vi "ALTS-2015 _Safety Logic LV2GBL.vi"(7 "Options":T1, 8 "error in (no error)":errorcluster, 10 "EStop In":bool) -> (0 "error out":errorcluster, 1 "S/W EStop":bool, 2 "EStop Out":bool, 3 "H/W EStop":bool)   [LabVIEW 2013]
uses:
  Controls/ALTS-2015 Safety Logic Cases.ctl
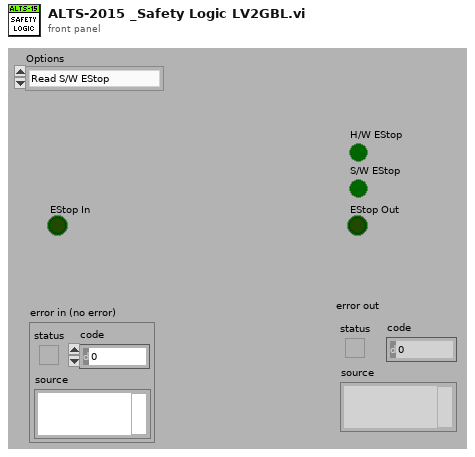
[diagram p1: front panel]
types:
  T1 = typedef "ALTS-2015 Safety Logic Cases.ctl" = enum16{"Read S/W EStop", "Read H/W EStop", "Write S/W EStop", "Write H/W EStop", "Read S/W & H/W EStop"}
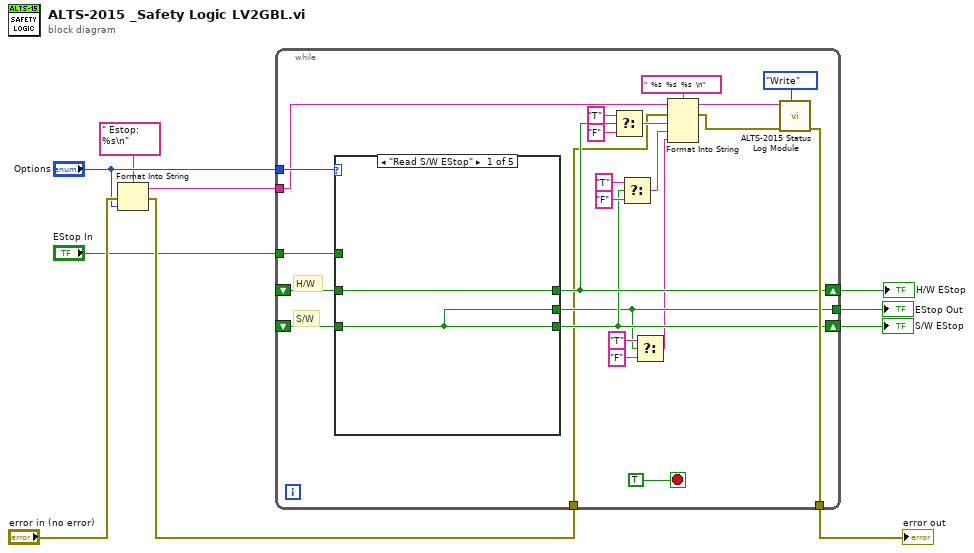
[diagram p0: block diagram]
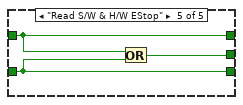
[diagram p5: hidden frame]
diagram:
  n1 = Format Into String(format string=" Estop: %s\n", error in="error in (no error)", "Options") -> (resulting string=w2:string, error out=w9:errorcluster)  [unwired: 1 in]
  n2 = while {
    shift-right: [w19] -> w5
    shift-left: _ -> [w32]
    tunnel: "Options" -> [w31]
    tunnel: "EStop In" -> [w30]
    shift-right: [w23] -> w6
    shift-left: _ -> [w29]
    tunnel: [w16] -> w7
    tunnel: w2 -> [w27]
    tunnel: [w34] -> w1
    tunnel: w9 -> [w12]
    stop <- TRUE stop-if-true
    # "H/W"
    # "S/W"
    n3 = case shown="\"Read S/W EStop\"" w31 {
      tunnel: w32 -> [w35 w37 _ w42 w43]
      tunnel: [w35 w37 w39 w42 w43] -> w19
      tunnel: w30 -> [_ _ w39 w41 _]
      tunnel: w29 -> [w36 w38 w40 _ w44]
      tunnel: [w36 w38 w40 w41 w44] -> w23
      tunnel: [w35 w38 w39 w41 w45] -> w16
      frame "Read S/W EStop" {
      }
      frame "Read H/W EStop" {
      }
      frame "Write S/W EStop" {
      }
      frame "Write H/W EStop" {
      }
      frame "Read S/W & H/W EStop" {
        n4 = Or(x=w44, y=w43) -> (x .or. y?=w45:bool)
      }
    }
    n5 = Select(t="T", s=w23, f="F") -> (s? t:f=w24:string)
    n6 = Select(t="T", s=w19, f="F") -> (s? t:f=w20:string)
    n7 = Select(t="T", s=w16, f="F") -> (s? t:f=w15:string)
    n8 = Format Into String(format string="  %s  %s  %s  \n", initial string=w27, error in=w12, w24, w20, w15) -> (resulting string=w14:string, error out=w11:errorcluster)
    n9 = call "ALTS-2015 Status Log Module.vi"("Options"=enum16{"Init", "Write", "Close"}."Write", "error in"=w11, "Text to  Log"=w14) -> ("error out"=w34:errorcluster)  [unwired: 8 in]
  }
  "error out" <- w1
  "EStop Out" <- w7
  "H/W EStop" <- w6
  "S/W EStop" <- w5
